vi "Exit Initialize (User).vi"(8 "error in":errorcluster, 11 "Node in":refnum<class "AMS Chiller Template.lvclass">) -> (0 "error out":errorcluster, 3 "Node out":refnum<class "AMS Chiller Template.lvclass">)   [LabVIEW 2023, in "AMS Chiller Template.lvlib" / "AMS Chiller Template.lvclass"]
uses:
  AMS Chiller Template.lvclass
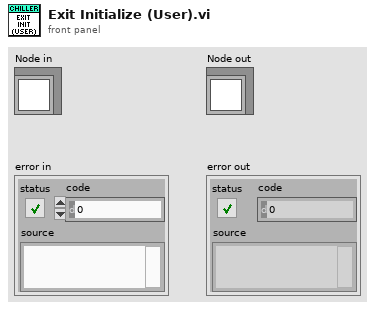
[diagram p1: front panel]
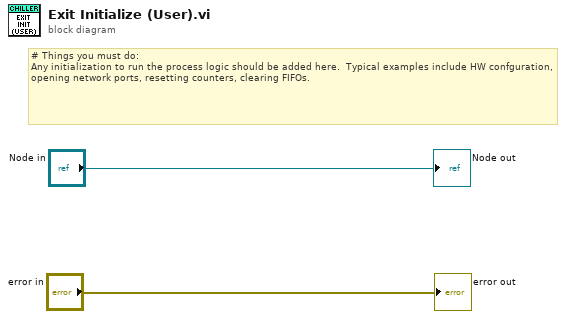
[diagram p0: block diagram]
diagram:
  # "# Things you must do:\nAny initialization to run the process logic should be added here.  Typical examples include HW confguration, opening network ports, resetting counters, clearing FIFOs."
  "Node out" <- "Node in"
  "error out" <- "error in"
